vi "Test.vi"() -> ()   [LabVIEW 2016]
uses:
  <vilib>/Utility/inputDevices.llb/mouseAcquire.vi
  <vilib>/Utility/inputDevices.llb/closeMouse.vi
  C:/Windows/System32/user32.dll
panel:
  out "point":T1
  out "return type 2":i32
  in  "rectClinet":T1
  out "axis info":T2
  out "Numeric":i32
  in  "stop":bool
  out "return type":i32 format="%x"
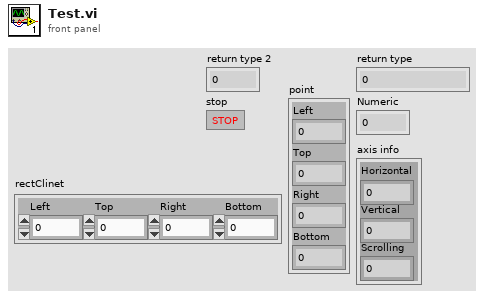
[diagram p1: front panel]
types:
  T1 = cluster{"Left":i32, "Top":i32, "Right":i32, "Bottom":i32}
  T2 = cluster{"Horizontal":i32, "Vertical":i32, "Scrolling":i32}
  T3 = cluster{"button 1":bool, "button 2":bool, "button 3":bool, "button 4":bool}
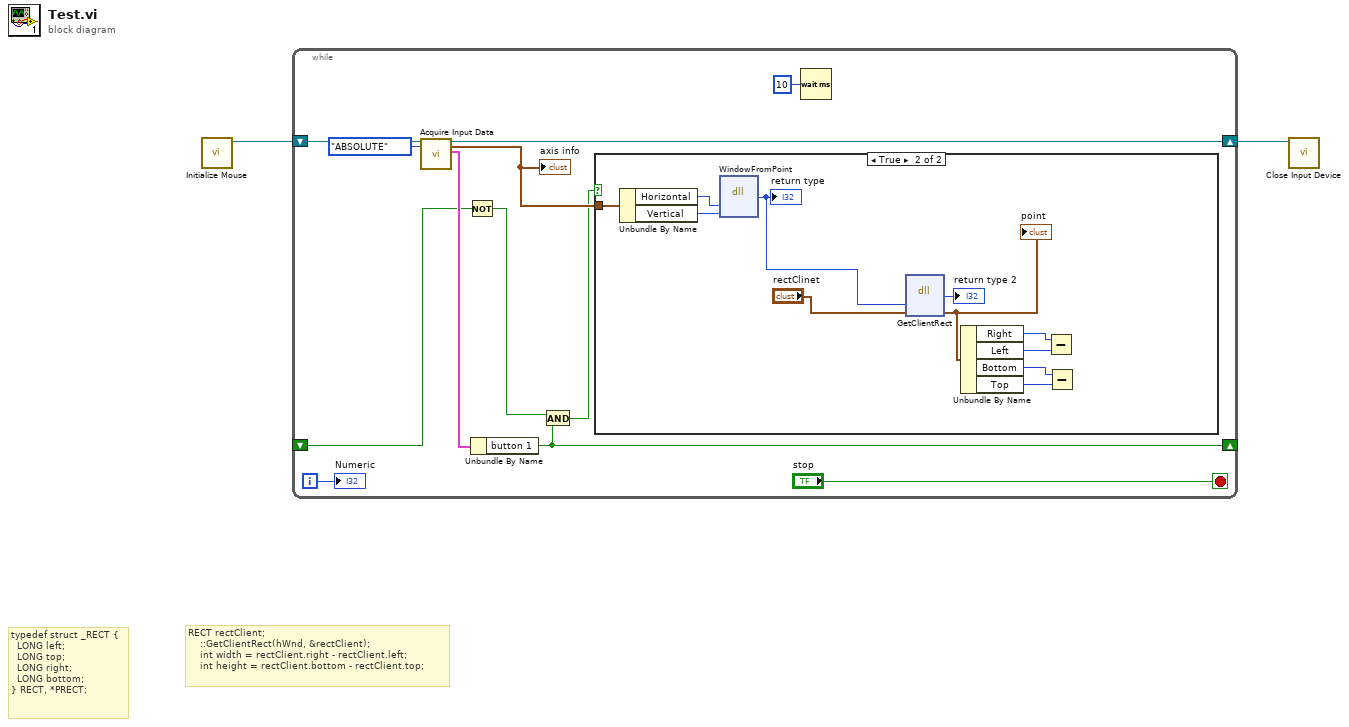
[diagram p0: block diagram]
diagram:
  # "typedef struct _RECT {\n  LONG left;\n  LONG top;\n  LONG right;\n  LONG bottom;\n} RECT, *PRECT;"
  # "RECT rectClient;  \n    ::GetClientRect(hWnd, &rectClient);  \n    int width = rectClient.right - rectClient.left;  \n    int height = rectClient.bottom - rectClient.top;"
  n1 = call <vilib>:"Initialize Mouse.vi"() -> ("device ID"=w2:refnum<k1>)  [unwired: 10 in, 1 out]
  n2 = while {
    shift-right: [w11] -> w1
    shift-left: w2 -> [w14]
    shift-right: [w8] -> _
    shift-left: _ -> [w9]
    i -> [w4]
    stop <- "stop" stop-if-true
    n3 = call-poly <vilib>:"Acquire Input Data.vi"("device ID"=w14, "key mode"=enum16{"RELATIVE", "ABSOLUTE"}."ABSOLUTE") -> ("device ID"=w11:refnum<k1>, "axis info"=w12:T2, "button info"=w10:T3)  [unwired: 14 in, 1 out]
    "axis info" <- w12
    n4 = Not(x=w9) -> (.not. x?=w7:bool)
    n5 = Unbundle By Name(w10) -> ("button 1"=w8:bool)
    n6 = And(x=w7, y=w8) -> (x .and. y?=w6:bool)
    n7 = case shown="True" w6 {
      tunnel: w12 -> [_ w25]
      frame False {
      }
      frame True {
        n8 = Unbundle By Name(w25) -> ("Horizontal"=w24:i32, "Vertical"=w23:i32)
        n9 = dll-call lib="C:/Windows/System32/user32.dll" fn="WindowFromPoint"("x"=w24, "y"=w23) -> ("return type"=w21:i32)  [unwired: 5 in, 2 out]
        "return type" <- w21
        n10 = dll-call lib="C:/Windows/System32/user32.dll" fn="GetClientRect"("HWND"=w21, "point"="rectClinet") -> ("return type"=→"return type 2":i32, "point"=w19:T1)  [unwired: 4 in, 2 out]
        "point" <- w19
        n11 = Unbundle By Name(w19) -> ("Right"=w17:i32, "Left"=w18:i32, "Bottom"=w16:i32, "Top"=w15:i32)
        n12 = Subtract(x=w17, y=w18) -> ()  [unwired: 1 out]
        n13 = Subtract(x=w16, y=w15) -> ()  [unwired: 1 out]
      }
    }
    n14 = Wait (ms)(milliseconds to wait=u32 10) -> ()  [unwired: 1 out]
    "Numeric" <- w4
  }
  n15 = call-poly <vilib>:"Close Input Device.vi"("device ID"=w1) -> ()  [unwired: 9 in, 1 out]
